vi "DriveAngleH.vi"(2 "Parameter String":string, 3 "Reinit":bool) -> (0 "Error Out":errorcluster, 1 "Increment":bool)   [LabVIEW 2020]
doc: "The swerve drive base will rotate about its center at a speed specified by the joystick command. This is a \"dumb\" algorithm, there is no feedback controller and the direction of rotation must be specified manually. Any complex or critical turns should be handled using either the Path Follower or auto-targeting. \n\nParameters:\n1. field-centric angle --> (deg) [0,360]\n2. relative rotation speed --> [-1,1]"
uses:
  SafeParser_Float.vi
  GlobalDriverStationCommands.vi
  GlobalPoseAndTargeting.vi
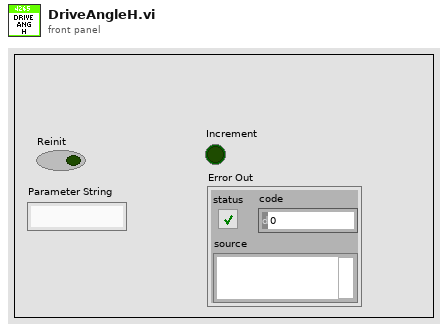
[diagram p1: front panel]
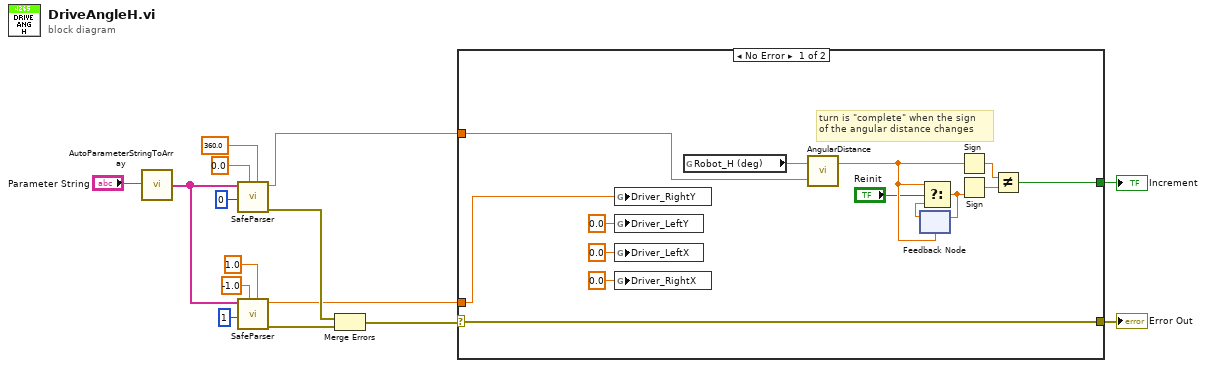
[diagram p0: block diagram]
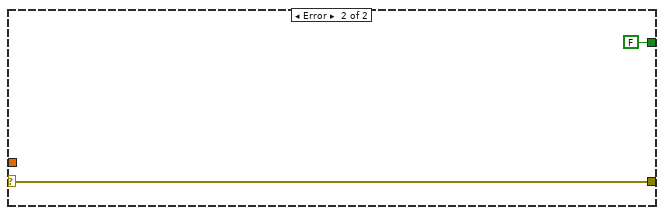
[diagram p2: hidden frame]
diagram:
  n1 = call "AutoParameterStringToArray.vi"("Parameter String"="Parameter String") -> ("Parsed Parameters"=w9:string[])
  n2 = call-poly "SafeParser.vi"("Maximum"=360.0, "Minimum"=0.0, "Array Index"=0 ("Parameter Index"), "String Array"=w9) -> ("Error Out"=w7:errorcluster, "Typecast  Value"=w5:dbl)  [unwired: 6 in]
  n3 = call-poly "SafeParser.vi"("Maximum"=1.0, "Minimum"=-1.0, "Array Index"=1 ("Parameter Index"), "String Array"=w9) -> ("Error Out"=w6:errorcluster, "Typecast  Value"=w4:dbl)  [unwired: 6 in]
  n4 = Merge Errors(w7, w6) -> (w8:errorcluster)
  n5 = case shown="No Error" w8 {
    selector: w8 -> [w20 w31]
    tunnel: [w16 FALSE] -> w1
    tunnel: [w20 w31] -> w15
    tunnel: w5 -> [w18 _]
    tunnel: w4 -> [w19 _]
    frame No Error {
      # "turn is \"complete\" when the sign\nof the angular distance changes"
      n6 = global write "GlobalDriverStationCommands.vi" "Driver_RightY"(w19) -> ()
      n7 = global write "GlobalDriverStationCommands.vi" "Driver_LeftY"(0.0 ("Driver_RightX")) -> ()
      n8 = global write "GlobalDriverStationCommands.vi" "Driver_LeftX"(0.0 ("Driver_RightX")) -> ()
      n9 = global write "GlobalDriverStationCommands.vi" "Driver_RightX"(0.0 ("Driver_RightX")) -> ()
      n10 = global read "GlobalPoseAndTargeting.vi" "Robot_H (deg)"() -> (w17:dbl)
      n11 = call "AngularDistance.vi"("Goal Angle (deg) [0,360]"=w18, "Current Angle (deg) [-Inf,+Inf]"=w17) -> ("Signed Angular Distance (deg) [-180,+180]"=w24:dbl)  [unwired: 1 out]
      n12 = feedback #1(w24) -> (w25:dbl)
      n13 = Select(t=w24, s="Reinit", f=w25) -> (s? t:f=w26:dbl)
      n14 = feedback-in #1(w26) -> ()
      n15 = Sign(1:w24) -> (0:w22:dbl)
      n16 = Sign(1:w26) -> (0:w23:dbl)
      n17 = Not Equal?(x=w22, y=w23) -> (x != y?=w16:bool)
    }
    frame Error {
    }
  }
  "Increment" <- w1
  "Error Out" <- w15
